vi "Enable EXFO Panel.vi"(8 "error in (no error)":errorcluster, 10 "Lock":bool, 11 "EXFO in":refnum<class "EXFO.lvclass">) -> (0 "error out":errorcluster, 3 "EXFO out":refnum<class "EXFO.lvclass">)   [LabVIEW 2018, in "EXFO.lvlib" / "EXFO.lvclass"]
doc: "This is the parent method VI, the child class will use the appropriate calls to lock or unlock the front panel controls on the EXFO to prevent technicians inadvertently changing the configurtation.\n\nAuthor: Ron Dexter\nCompany: Luminar\nModified: 5/20/2018"
uses:
  EXFO.lvclass
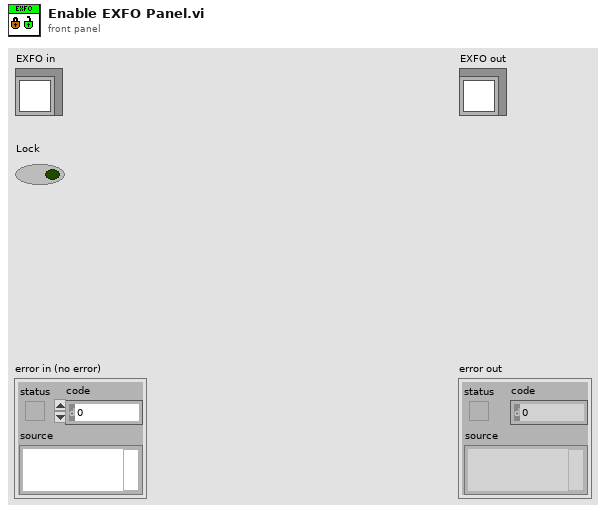
[diagram p1: front panel]
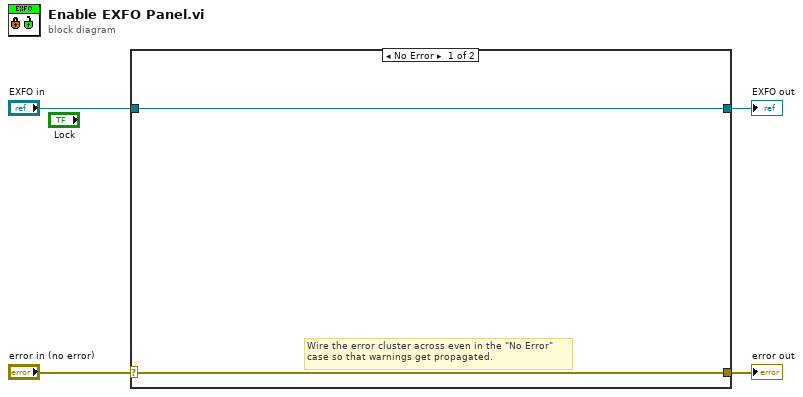
[diagram p0: block diagram]
diagram:
  n1 = case shown="No Error" "error in (no error)" {
    selector: "error in (no error)" -> [w5 w8]
    tunnel: [w5 w8] -> w3
    tunnel: [w6 w7] -> w1
    tunnel: "EXFO in" -> [w6 w7]
    frame No Error {
      # "Wire the error cluster across even in the \"No Error\"\ncase so that warnings get propagated."
    }
    frame Error {
    }
  }
  "error out" <- w3
  "EXFO out" <- w1
